vi "SearchArrayPathWrap.vi"(6 "Current Direction (T=Positive)":bool=TRUE, 9 "Target":T3, 10 "Current Pos":T2, 11 "All Lines":T4) -> (1 "Found Path?":bool, 2 "Path taken out":T1[][](array[typedef]))   [LabVIEW 2014, in "Map Data.lvlib"]
uses:
  Map Data.lvlib
  All-Lines.ctl
  LineCluster.ctl
  LineConnection.ctl
  Components/PathFinder/Controls/PathControl.ctl
panel:
  in  "Path Taken":T1[](array[typedef])
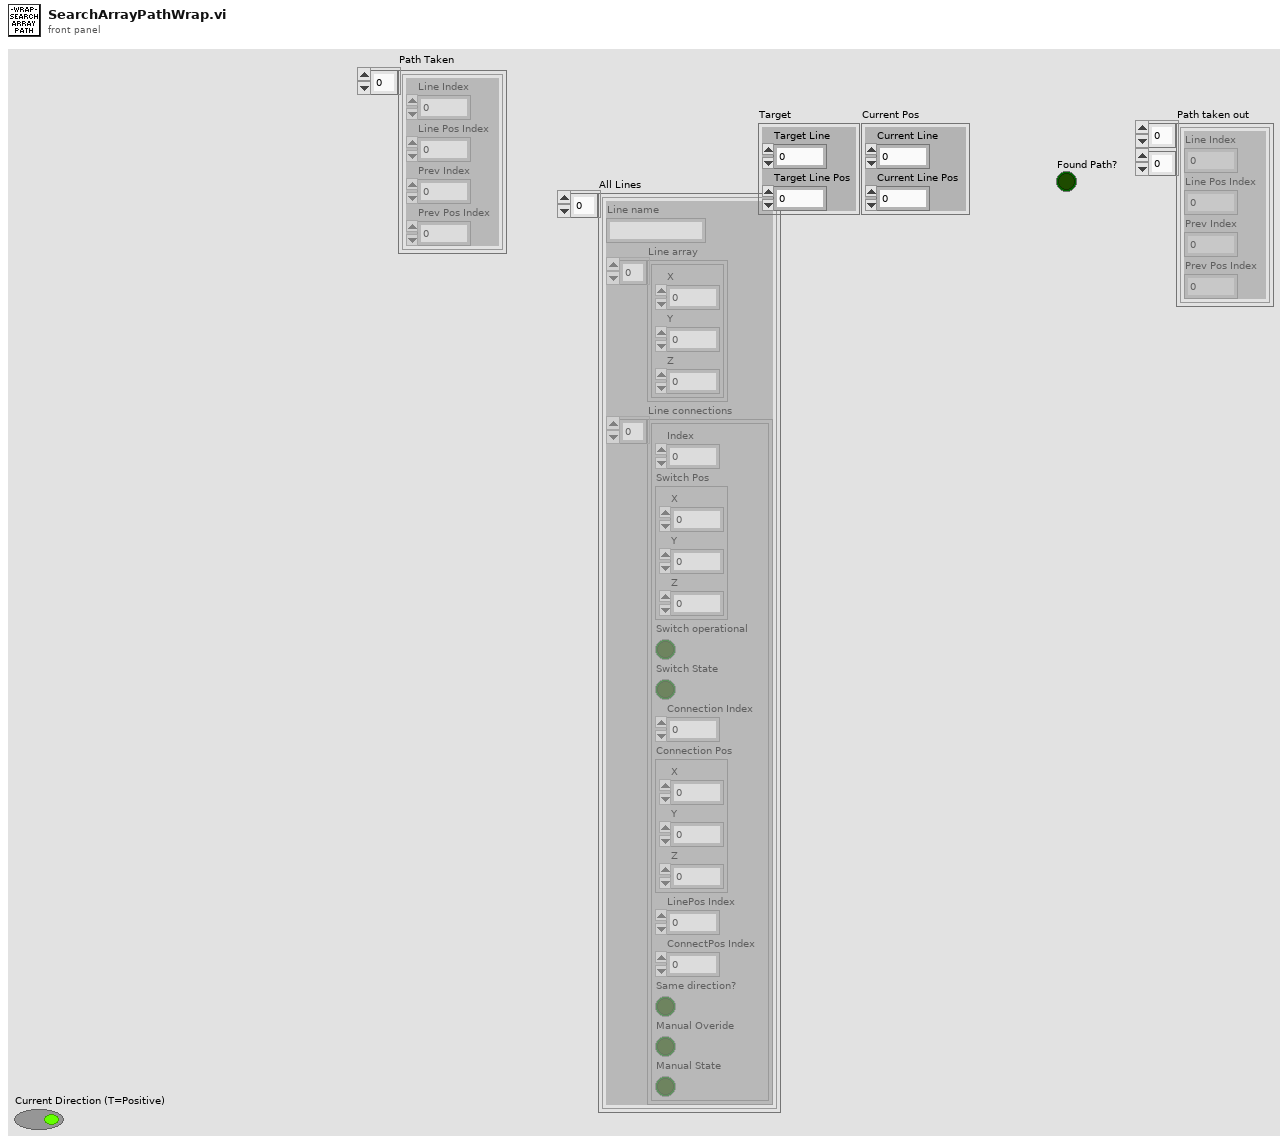
[diagram p1: front panel]
types:
  T1 = typedef "PathControl.ctl" = cluster{"Line Index":i32, "Line Pos Index ":i32, "Prev Index ":i32, "Prev Pos Index":i32}
  T2 = cluster{"Current Line":i32, "Current Line Pos":i32}
  T3 = cluster{"Target Line":i32, "Target Line Pos":i32}
  T4 = typedef "Map Data.lvlib/All-Lines.ctl" = T5[]
  T5 = typedef "Map Data.lvlib/LineCluster.ctl" = cluster{"Line name":string, "Line array":cluster{"X":dbl, "Y":dbl, "Z":dbl}[], "Line connections":T6[]}
  T6 = typedef "LineConnection.ctl" = cluster{"Index":i32, "Switch Pos":cluster{"X":dbl, "Y":dbl, "Z":dbl}, "Switch operational":bool, "Switch State":bool, "Connection Index":i32, "Connection Pos":cluster{"X":dbl, "Y":dbl, "Z":dbl}, "LinePos Index":i32, "ConnectPos Index":i32, "Same direction?":bool, "Manual Overide":bool, "Manual State":bool}
  T7 = cluster{"Target Line":i32, "Target Line Pos":i32, "Target Line Pos":i32, "Target Line Pos":i32}
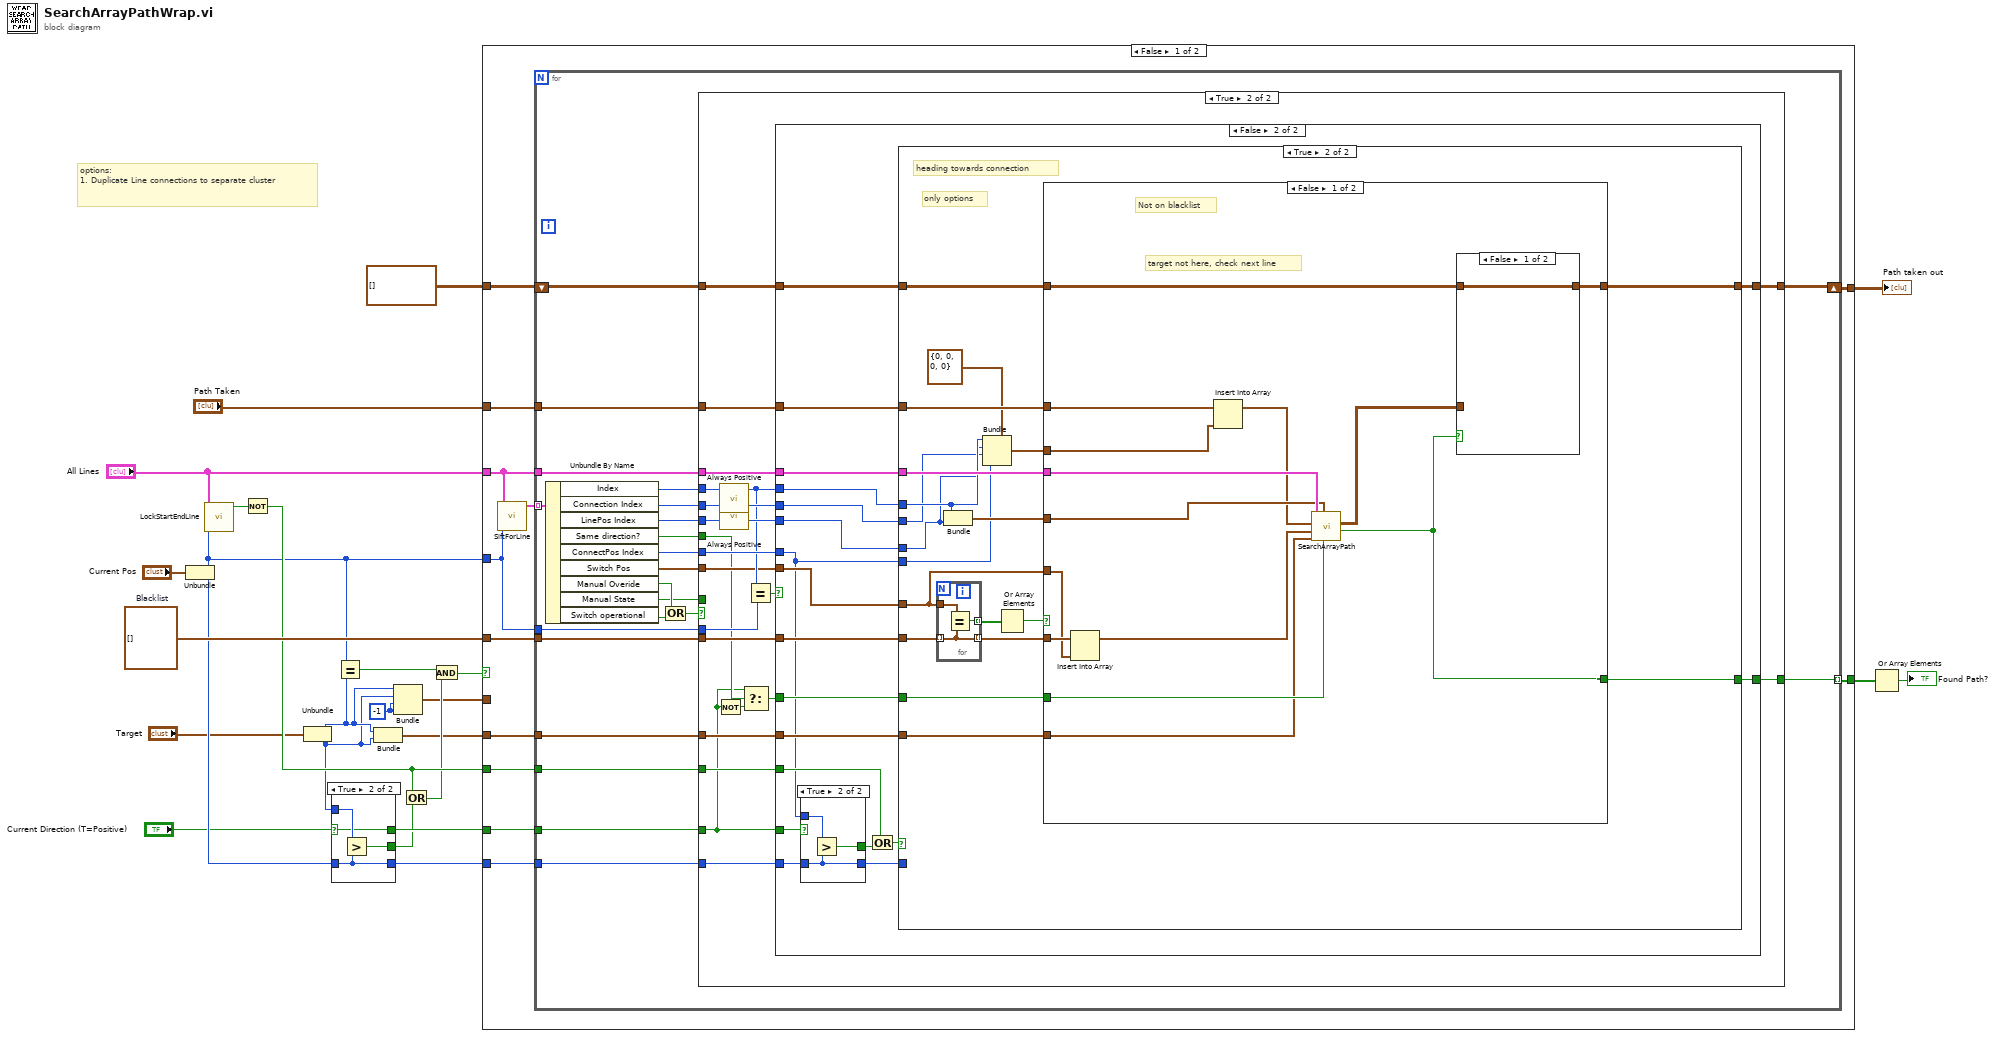
[diagram p0: block diagram]
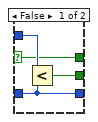
[diagram p2: hidden frame]
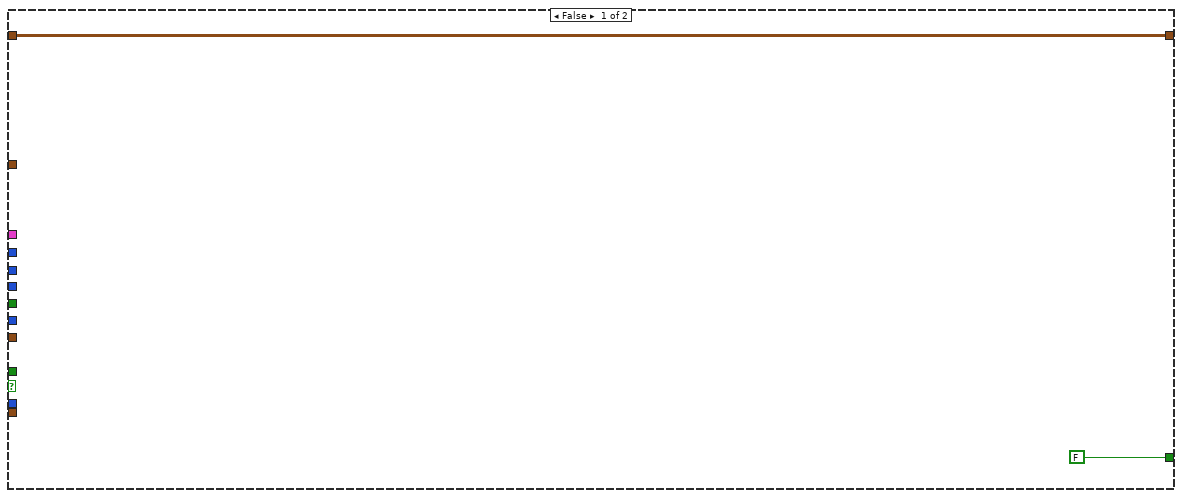
[diagram p3: hidden frame]
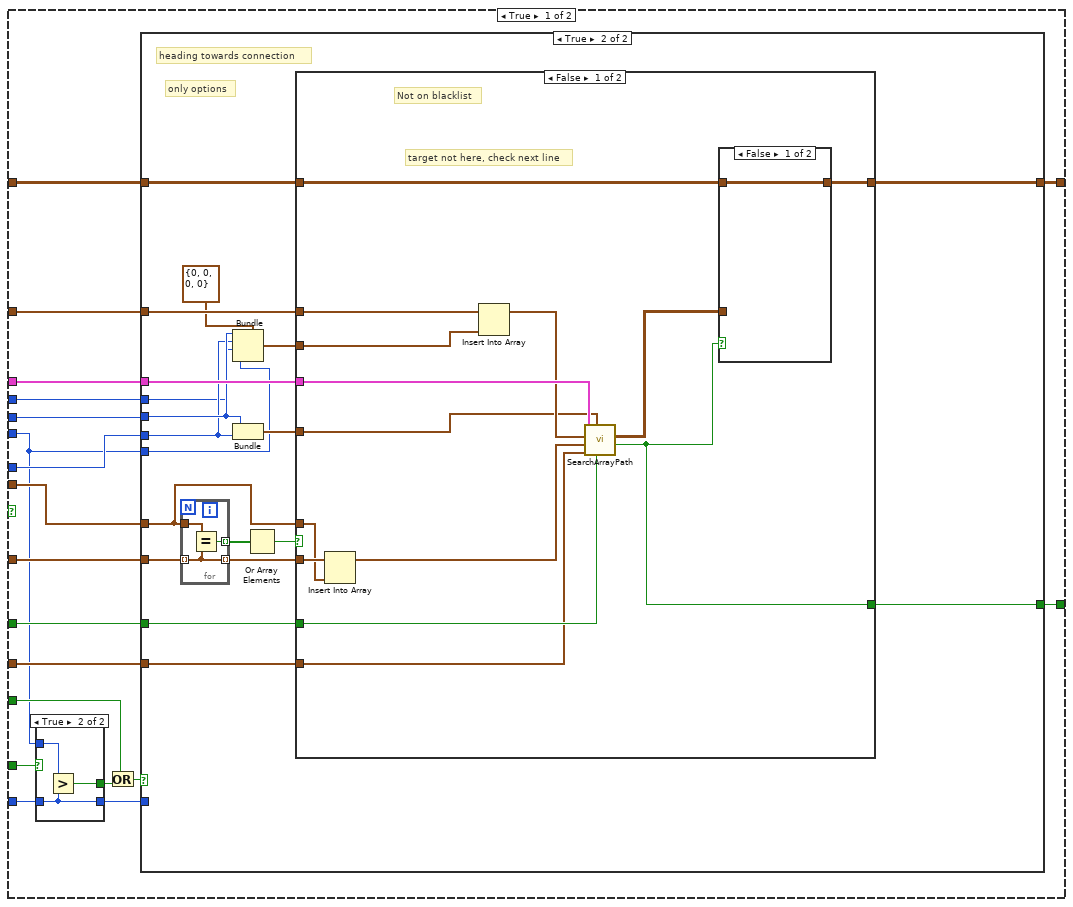
[diagram p4: hidden frame]
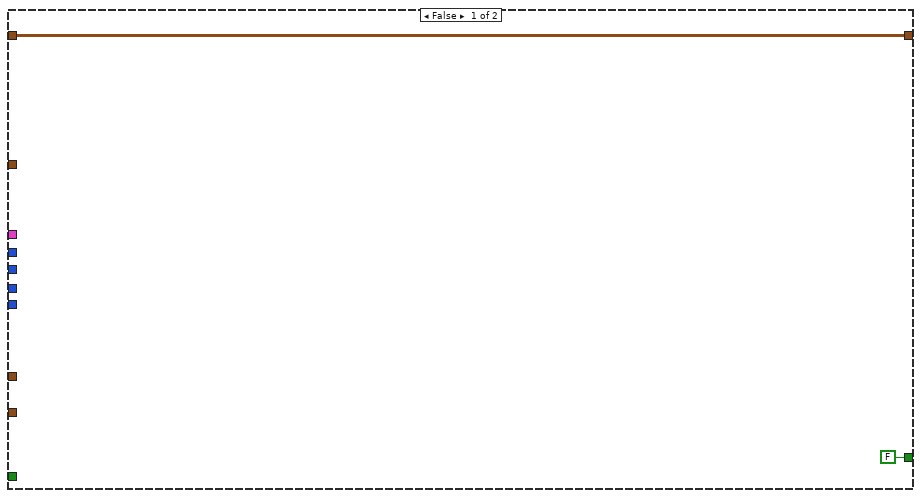
[diagram p5: hidden frame]
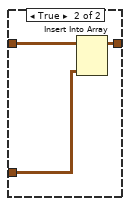
[diagram p6: hidden frame]
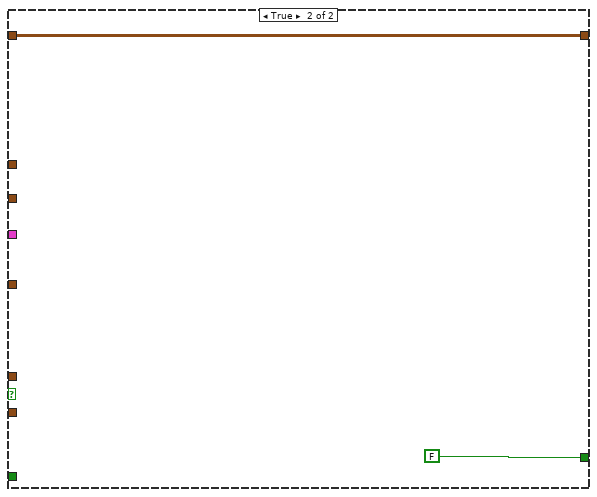
[diagram p7: hidden frame]
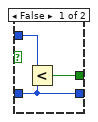
[diagram p8: hidden frame]
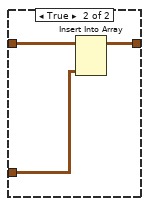
[diagram p10: hidden frame]
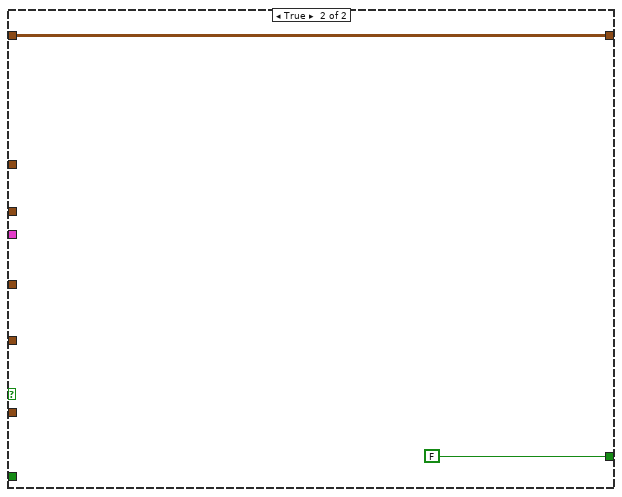
[diagram p11: hidden frame]
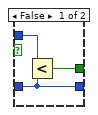
[diagram p12: hidden frame]
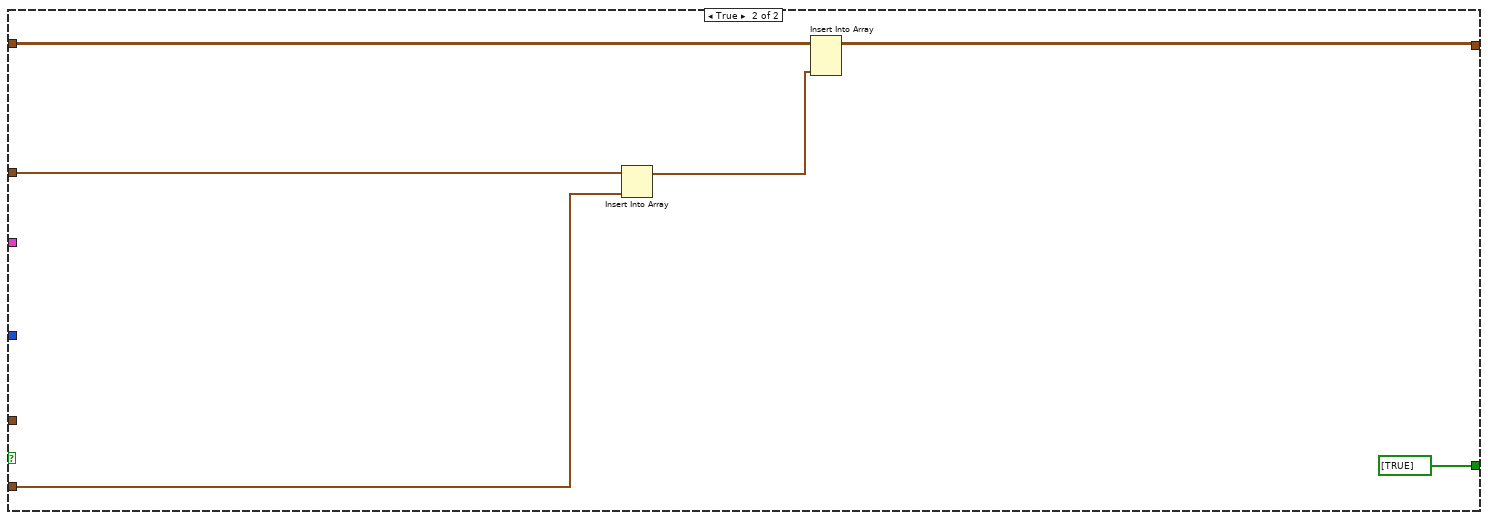
[diagram p13: hidden frame]
diagram:
  w3 = -1 ("Target Line Pos")
  w24 = cluster{"X":dbl, "Y":dbl, "Z":dbl}[] []  # Blacklist
  # "options: \n1. Duplicate Line connections to separate cluster"
  n1 = Unbundle("Current Pos") -> ("Current Line"=w1:i32, "Current Line Pos"=w18:i32)
  n2 = call "LockStartEndLine.vi"("index"=w1, "All Lines"="All Lines") -> ("Not Locked?"=w20:bool)  [unwired: 9 in]
  n3 = Not(x=w20) -> (.not. x?=w13:bool)
  n4 = Unbundle("Target") -> ("Target Line"=w5:i32, "Target Line Pos"=w4:i32)
  n5 = case shown="True" "Current Direction (T=Positive)" {
    selector: "Current Direction (T=Positive)" -> [w27 w31]
    tunnel: w4 -> [w29 w33]
    tunnel: w18 -> [w26 w30]
    tunnel: [w28 w32] -> w14
    tunnel: [w27 w31] -> w15
    tunnel: [w26 w30] -> w17
    frame False {
      n6 = Less?(x=w29, y=w26) -> (x < y?=w28:bool)
    }
    frame True {
      n7 = Greater?(x=w33, y=w30) -> (0:w32:bool)
    }
  }
  n8 = Equal?(x=w1, y=w5) -> (x = y?=w12:bool)
  n9 = Bundle("Target Line"=w5, "Target Line Pos"=w4) -> (w8:T3)  [unwired: 1 in]
  n10 = Bundle("Target Line"=w5, "Target Line Pos"=w4, "Target Line Pos"=w3, "Target Line Pos"=w3) -> (w2:T7)  [unwired: 1 in]
  n11 = Or(x=w13, y=w14) -> (x .or. y?=w11:bool)
  n12 = And(x=w12, y=w11) -> (x .and. y?=w10:bool)
  n13 = case shown="False" w10 {
    tunnel: w15 -> [w45 _]
    tunnel: w17 -> [w44 _]
    tunnel: "Path Taken" -> [w43 w235]
    tunnel: w24 -> [w42 _]
    tunnel: T1[][] [] ("Path taken") -> [w41 w234]
    tunnel: [w40 w232] -> w6
    tunnel: [w39 bool[] [TRUE]] -> w21
    tunnel: w13 -> [w38 _]
    tunnel: "All Lines" -> [w37 _]
    tunnel: w8 -> [w34 _]
    tunnel: w2 -> [_ w230]
    tunnel: w1 -> [w35 _]
    frame False {
      n14 = call "SiftForLine.vi"("Current Line"=w35, "All Lines"=w37) -> ("Line connections"=w36:T6[])  [unwired: 9 in]
      n15 = for {
        tunnel: w36 -> [w65] mode=indexing
        tunnel: w42 -> [w66]
        tunnel: [w63] -> w39 mode=indexing
        tunnel: w37 -> [w64]
        tunnel: w43 -> [w67]
        tunnel: w45 -> [w50]
        tunnel: w44 -> [w62]
        shift-right: [w59] -> w40
        shift-left: w41 -> [w58]
        tunnel: w38 -> [w57]
        tunnel: w35 -> [w54]
        tunnel: w34 -> [w52]
        n16 = Unbundle By Name(w65) -> ("Index"=w56:i32, "Connection Index"=w55:i32, "LinePos Index"=w61:i32, "Same direction?"=w51:bool, "ConnectPos Index"=w60:i32, "Switch Pos"=w53:cluster{"X":dbl, "Y":dbl, "Z":dbl}, "Manual Overide"=w49:bool, "Manual State"=w46:bool, "Switch operational"=w48:bool)
        n17 = Or(x=w49, y=w48) -> (x .or. y?=w47:bool)
        n18 = case shown="True" w47 {
          tunnel: w67 -> [_ w91]
          tunnel: w66 -> [_ w90]
          tunnel: w64 -> [_ w89]
          tunnel: [FALSE ("Found Path?") w88] -> w63
          tunnel: w62 -> [_ w87]
          tunnel: w61 -> [_ w86]
          tunnel: w60 -> [_ w85]
          tunnel: [w69 w84] -> w59
          tunnel: w58 -> [w69 w83]
          tunnel: w57 -> [_ w82]
          tunnel: w56 -> [_ w81]
          tunnel: w55 -> [_ w80]
          tunnel: w54 -> [_ w78]
          tunnel: w53 -> [_ w76]
          tunnel: w52 -> [_ w74]
          tunnel: w51 -> [_ w73]
          tunnel: w50 -> [_ w72]
          tunnel: w46 -> [_ _]
          frame False {
          }
          frame True {
            n19 = Not(x=w72) -> (.not. x?=w70:bool)
            n20 = call "Always Positive.vi"("Input"=w81) -> ("Output"=w77:i32)  [unwired: 8 in]
            n21 = call "Always Positive.vi"("Input"=w80) -> ("Output"=w79:i32)  [unwired: 8 in]
            n22 = Select(t=w72, s=w73, f=w70) -> (s? t:f=w71:bool)
            n23 = Equal?(x=w77, y=w78) -> (x = y?=w75:bool)
            n24 = case shown="False" w75 {
              tunnel: w91 -> [w110 w179]
              tunnel: w90 -> [w109 w178]
              tunnel: w89 -> [w108 w177]
              tunnel: [w107 w176] -> w88
              tunnel: w72 -> [w106 w175]
              tunnel: w87 -> [w105 w174]
              tunnel: w86 -> [w92 w165]
              tunnel: w76 -> [w103 w172]
              tunnel: w85 -> [w102 w161]
              tunnel: [w101 w171] -> w84
              tunnel: w83 -> [w100 w170]
              tunnel: w82 -> [w98 w168]
              tunnel: w79 -> [w96 w164]
              tunnel: w77 -> [w95 w166]
              tunnel: w74 -> [w94 w163]
              tunnel: w71 -> [w93 w162]
              frame True {
                n25 = case shown="True" w106 {
                  tunnel: w92 -> [w156 w159]
                  tunnel: w105 -> [w155 w158]
                  tunnel: [w157 w160] -> w99
                  tunnel: [w155 w158] -> w104
                  frame False {
                    n26 = Less?(x=w156, y=w155) -> (x < y?=w157:bool)
                  }
                  frame True {
                    n27 = Greater?(x=w159, y=w158) -> (0:w160:bool)
                  }
                }
                n28 = Or(x=w98, y=w99) -> (x .or. y?=w97:bool)
                n29 = case shown="True" w97 {
                  tunnel: w110 -> [_ w131]
                  tunnel: w96 -> [_ w116]
                  tunnel: w109 -> [_ w129]
                  tunnel: w108 -> [_ w128]
                  tunnel: [FALSE ("Found Path?") w127] -> w107
                  tunnel: w104 -> [_ _]
                  tunnel: w103 -> [_ w121]
                  tunnel: w102 -> [_ w115]
                  tunnel: [w111 w123] -> w101
                  tunnel: w100 -> [w111 w122]
                  tunnel: w95 -> [_ w114]
                  tunnel: w94 -> [_ w120]
                  tunnel: w93 -> [_ w119]
                  tunnel: w92 -> [_ w113]
                  frame False {
                  }
                  frame True {
                    # "only options"
                    # "heading towards connection"
                    n30 = for {
                      tunnel: w129 -> [w134] mode=indexing
                      tunnel: w121 -> [w132]
                      tunnel: [w133] -> w126 mode=indexing
                      tunnel: [w134] -> w125 mode=indexing
                      n31 = Equal?(x=w132, y=w134) -> (x = y?=w133:bool)
                    }
                    n32 = Bundle(cluster=T1 {"Line Index"=0, "Line Pos Index "=0, "Prev Index "=0, "Prev Pos Index"=0} ("Posits"), "Line Index"=w116, "Line Pos Index"=w115, "Prev Index"=w114, "Prev Pos Index"=w113) -> (w117:T1)
                    n33 = Bundle("Output"=w116, "ConnectPos Index"=w115) -> (w124:cluster{"Output":i32, "ConnectPos Index":i32})  [unwired: 1 in]
                    n34 = Or Array Elements(Boolean array=w126) -> (logical OR=w130:bool)
                    n35 = case shown="False" w130 {
                      tunnel: w131 -> [w148 _]
                      tunnel: w125 -> [w145 _]
                      tunnel: w120 -> [w137 _]
                      tunnel: [w147 FALSE] -> w127
                      tunnel: w128 -> [w146 _]
                      tunnel: w121 -> [w143 _]
                      tunnel: w124 -> [w135 _]
                      tunnel: [w142 w153] -> w123
                      tunnel: w122 -> [w141 w153]
                      tunnel: w119 -> [w138 _]
                      tunnel: w117 -> [w136 _]
                      frame False {
                        # "target not here, check next line"
                        # "Not on blacklist"
                        n36 = Insert Into Array(array=w145, new element=w143) -> (w144:cluster{"X":dbl, "Y":dbl, "Z":dbl}[])  [unwired: 1 in]
                        n37 = Insert Into Array(array=w148, new element=w136) -> (w140:T1[])  [unwired: 1 in]
                        n38 = call "SearchArrayPath.vi"("Current Direction (T=Positive)"=w138, "Current Pos"=w135, "Target"=w137, "Blacklist"=w144, "Path Taken"=w140, "All Lines"=w146) -> ("Found Path?"=w147:bool, "Path taken"=w139:T1[][])  [unwired: 4 in]
                        n39 = case shown="False" w147 {
                          tunnel: w139 -> [_ w150]
                          tunnel: w141 -> [w149 w152]
                          tunnel: [w149 w151] -> w142
                          frame False {
                          }
                          frame True {
                            n40 = Insert Into Array(array=w152, new element=w150) -> (w151:T1[][])  [unwired: 2 in]
                          }
                        }
                      }
                      frame True {
                      }
                    }
                  }
                }
              }
              frame False {
                n41 = case shown="True" w175 {
                  tunnel: w161 -> [w225 w228]
                  tunnel: w174 -> [w224 w227]
                  tunnel: [w226 w229] -> w169
                  tunnel: [w224 w227] -> w173
                  frame False {
                    n42 = Less?(x=w225, y=w224) -> (x < y?=w226:bool)
                  }
                  frame True {
                    n43 = Greater?(x=w228, y=w227) -> (0:w229:bool)
                  }
                }
                n44 = Or(x=w168, y=w169) -> (x .or. y?=w167:bool)
                n45 = case shown="True" w167 {
                  selector: w167 -> [w180 _]
                  tunnel: w179 -> [_ w200]
                  tunnel: w166 -> [_ w185]
                  tunnel: w178 -> [_ w198]
                  tunnel: w177 -> [_ w197]
                  tunnel: [w180 w196] -> w176
                  tunnel: w173 -> [_ _]
                  tunnel: w172 -> [_ w189]
                  tunnel: w162 -> [_ w193]
                  tunnel: w165 -> [_ w184]
                  tunnel: [w181 w191] -> w171
                  tunnel: w170 -> [w181 w190]
                  tunnel: w164 -> [_ w183]
                  tunnel: w163 -> [_ w188]
                  tunnel: w161 -> [_ w182]
                  frame False {
                  }
                  frame True {
                    # "only options"
                    # "heading towards connection"
                    n46 = for {
                      tunnel: w198 -> [w203] mode=indexing
                      tunnel: w189 -> [w201]
                      tunnel: [w202] -> w195 mode=indexing
                      tunnel: [w203] -> w194 mode=indexing
                      n47 = Equal?(x=w201, y=w203) -> (x = y?=w202:bool)
                    }
                    n48 = Bundle("Output"=w185, "LinePos Index"=w184) -> (w192:cluster{"Output":i32, "LinePos Index":i32})  [unwired: 1 in]
                    n49 = Bundle(cluster=T1 {"Line Index"=0, "Line Pos Index "=0, "Prev Index "=0, "Prev Pos Index"=0} ("Posits"), "Line Index"=w185, "Line Pos Index"=w184, "Prev Index"=w183, "Prev Pos Index"=w182) -> (w186:T1)
                    n50 = Or Array Elements(Boolean array=w195) -> (logical OR=w199:bool)
                    n51 = case shown="False" w199 {
                      tunnel: w200 -> [w217 _]
                      tunnel: w194 -> [w214 _]
                      tunnel: w188 -> [w205 _]
                      tunnel: [w216 FALSE] -> w196
                      tunnel: w197 -> [w215 _]
                      tunnel: w189 -> [w212 _]
                      tunnel: w193 -> [w211 _]
                      tunnel: w192 -> [w210 _]
                      tunnel: [w209 w222] -> w191
                      tunnel: w190 -> [w208 w222]
                      tunnel: w186 -> [w204 _]
                      frame False {
                        # "target not here, check next line"
                        # "Not on blacklist"
                        n52 = Insert Into Array(array=w214, new element=w212) -> (w213:cluster{"X":dbl, "Y":dbl, "Z":dbl}[])  [unwired: 1 in]
                        n53 = Insert Into Array(array=w217, new element=w204) -> (w207:T1[])  [unwired: 1 in]
                        n54 = call "SearchArrayPath.vi"("Current Direction (T=Positive)"=w211, "Current Pos"=w210, "Target"=w205, "Blacklist"=w213, "Path Taken"=w207, "All Lines"=w215) -> ("Found Path?"=w216:bool, "Path taken"=w206:T1[][])  [unwired: 4 in]
                        n55 = case shown="False" w216 {
                          tunnel: w206 -> [_ w219]
                          tunnel: w208 -> [w218 w221]
                          tunnel: [w218 w220] -> w209
                          frame False {
                          }
                          frame True {
                            n56 = Insert Into Array(array=w221, new element=w219) -> (w220:T1[][])  [unwired: 2 in]
                          }
                        }
                      }
                      frame True {
                      }
                    }
                  }
                }
              }
            }
          }
        }
      }
    }
    frame True {
      n57 = Insert Into Array(array=w235, new element=w230) -> (w233:T1[])  [unwired: 1 in]
      n58 = Insert Into Array(array=w234, new element=w233) -> (w232:T1[][])  [unwired: 2 in]
    }
  }
  "Path taken out" <- w6
  n59 = Or Array Elements(Boolean array=w21) -> (logical OR=→"Found Path?":bool)
